vi "Network Settings Viewer_.vi"() -> ()   [LabVIEW 2015]
doc: "Displays network settings for network adapters on specified target. Target must have \"NI System Configuration Remote Support\" installed to correctly obtain all settings."
uses:
  <vilib>/nisyscfg/Access Point.ctl
  <vilib>/nisyscfg/Wireless Network.ctl
  <vilib>/Utility/error.llb/DialogType.ctl
  <vilib>/nisyscfg/Close (Hardware).vi
  <vilib>/nisyscfg/Close (Filter).vi
  <vilib>/nisyscfg/Close (System).vi
  <vilib>/nisyscfg/nisyscfg.lvlib
  <resource>/objmgr/nisysapi.rc
panel:
  in  "Timeout (milliseconds)":u32=5000
  in  "User Name":string
  in  "Password":string
  in  "Target":refnum<k21>="localhost"
  in  "Network Settings":enum32{"Ethernet", "WLAN", "WLAN Access Points"}(tab)
  out "Ethernet":string[][](table)
  out "WLAN":string[][](table) caption="Ethernet"
  out "Access Points":T1[](array[typedef]) {"wireless network"."security type" items=["none"=0, "open"=2, "WEP"=4, "WPA Personal"=8, "WPA Enterprise"=16, "WPA2 Personal"=32, "WPA2 Enterprise"=64]; "wireless network"."connection type" items=["none", "infrastructure", "ad hoc"]; "link speed" items=["none"=0, "autonegotiate"=1, "10mbps/Half Duplex"=2, "10mbps/Full Duplex"=4, "100mbps/Half Duplex"=8, "100mbps/Full Duplex"=16, "Gigabit/Half Duplex"=32, "Gigabit/Full Duplex"=64, "WLAN 802.11a"=131072, "WLAN 802.11b"=262144, "WLAN 802.11g"=524288, "WLAN 802.11n"=1048576, "WLAN 802.11n (5GHz)"=2097152]}
  # "Overview: Displays network settings for network adapters on specified target.\nRequirements: NI System Configuration\nInstructions:\n1. Select Target. Enter User Name and Password if necessary.\n2. Run the VI."
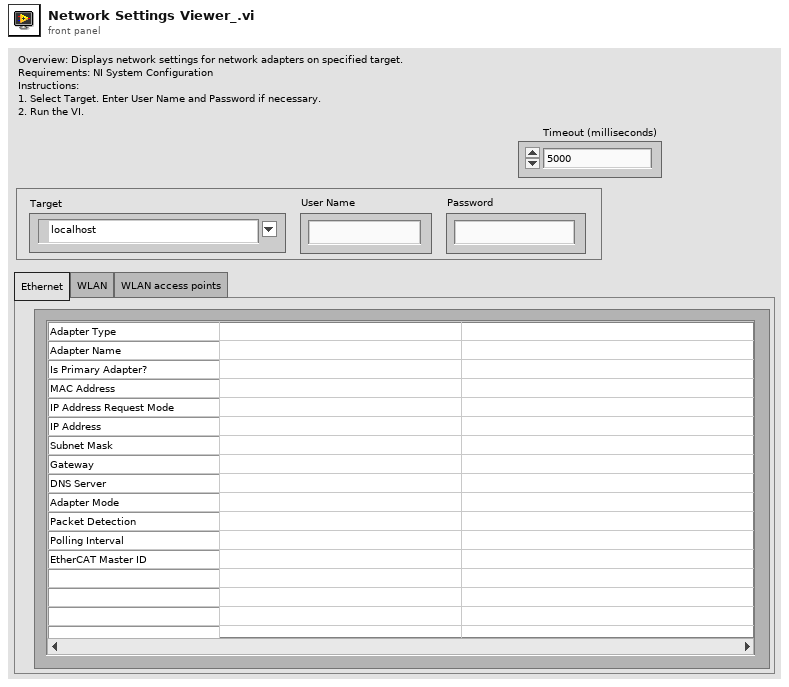
[diagram p1: front panel]
types:
  T1 = typedef "nisyscfg.lvlib/Access Point.ctl" = cluster{"wireless network":T2, "BSSID":string, "link quality":u32, "channel number":u32, "link speed":u32}
  T2 = typedef "nisyscfg.lvlib/Wireless Network.ctl" = cluster{"SSID":string, "connection type":u32, "security type":u32}
  T3 = typedef "DialogType.ctl" = u16
  T4 = typedef "Access Point.ctl" = cluster{"wireless network":T2, "BSSID":string, "link quality":u32, "channel number":u32, "link speed":u32}
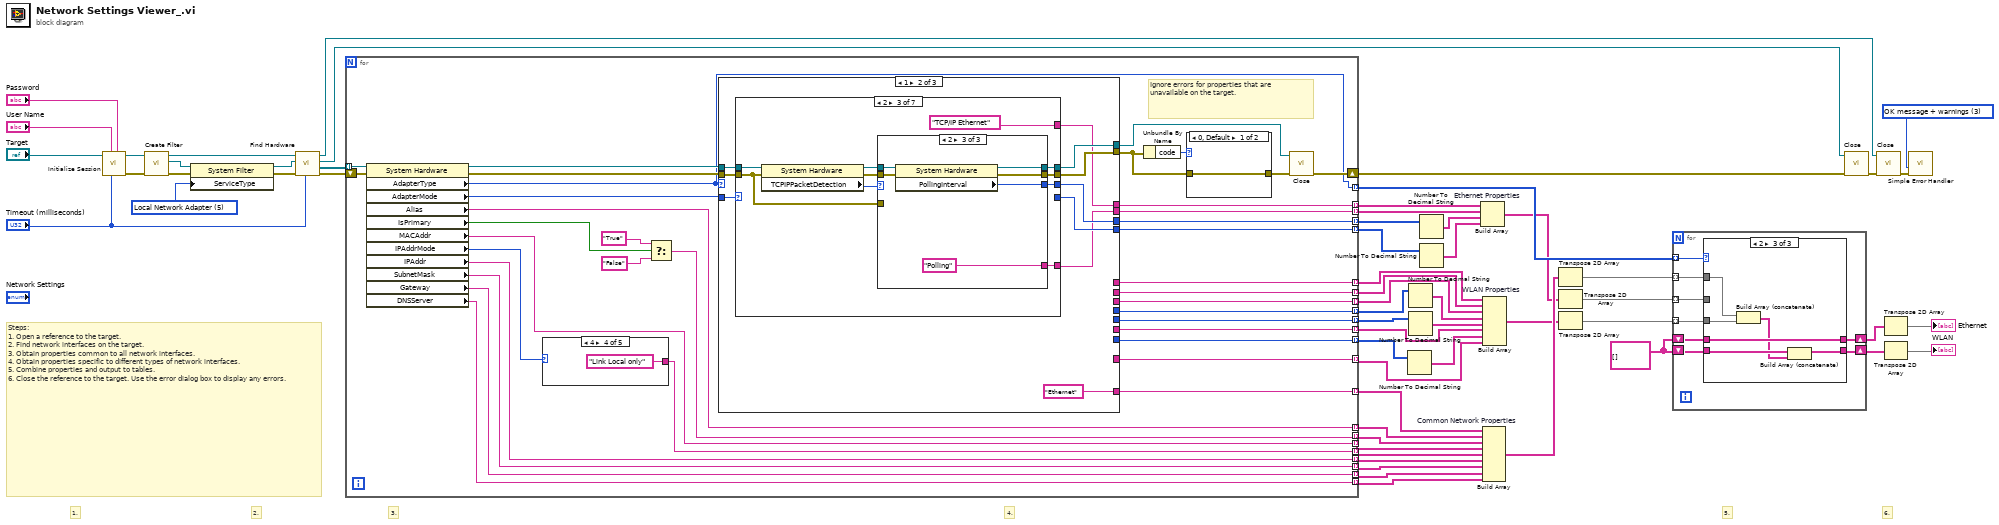
[diagram p0: block diagram]
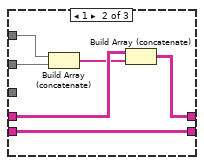
[diagram p3: hidden frame]
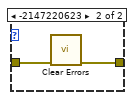
[diagram p4: hidden frame]
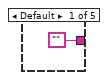
[diagram p5: hidden frame]
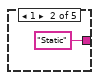
[diagram p6: hidden frame]
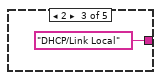
[diagram p7: hidden frame]
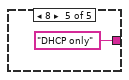
[diagram p8: hidden frame]
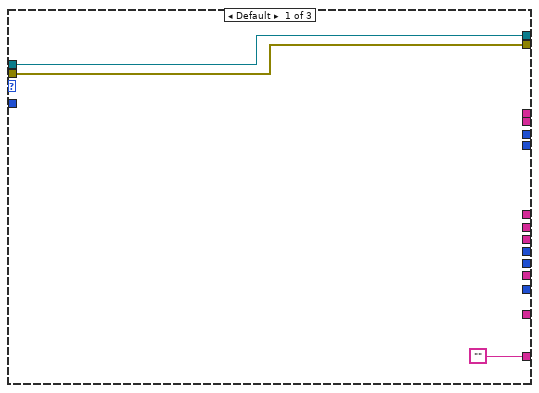
[diagram p9: hidden frame]
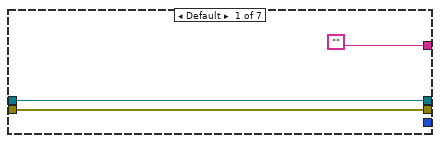
[diagram p10: hidden frame]
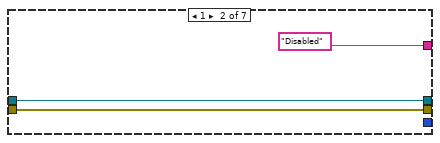
[diagram p11: hidden frame]
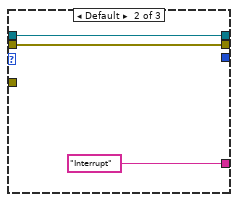
[diagram p13: hidden frame]
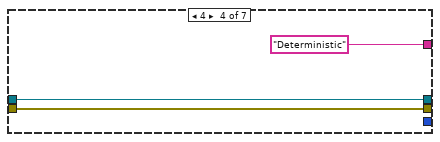
[diagram p14: hidden frame]
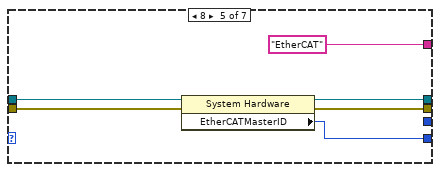
[diagram p15: hidden frame]
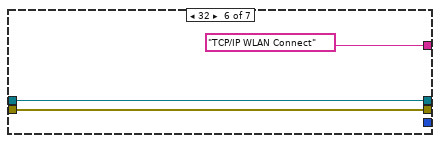
[diagram p16: hidden frame]
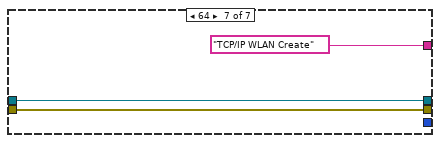
[diagram p17: hidden frame]
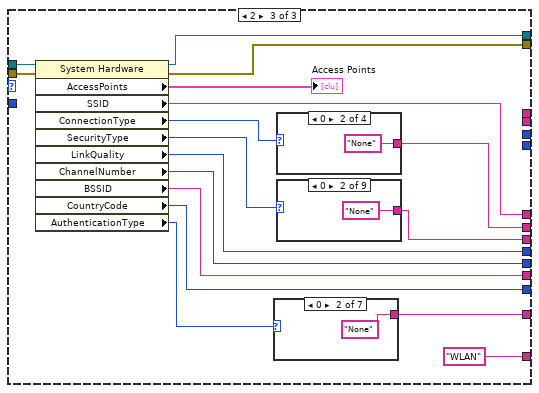
[diagram p18: hidden frame]
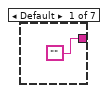
[diagram p19: hidden frame]
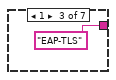
[diagram p20: hidden frame]
diagram:
  w3 = u32 5 items=["NI Network Resource", "NI Real-Time", "NI System Configuration", "NI Web Interface", "Local System", "Local Network Adapter", "Local Time Keeper", "Local Time Reference", "LXI Instrument"] ("Service Type")
  w4 = string[][] []
  w11 = T3 3 items=["no dialog", "OK message", "continue or stop message", "OK message + warnings", "continue/stop + warnings"] ("type of dialog (OK msg:1)")
  # "3."
  # "Steps:\n1. Open a reference to the target.\n2. Find network interfaces on the target.\n3. Obtain properties common to all network interfaces.\n4. Obtain properties specific to different types of network interfaces.\n5. Combine properties and output to tables.\n6. Close the reference to the target. Use the error dialog box to display any errors."
  # "6."
  # "5."
  # "4."
  # "2."
  # "1."
  n1 = call <vilib>:"Initialize Session.vi"("Password"="Password", "Connect Timeout (4000 ms)"="Timeout (milliseconds)", "User Name"="User Name", "Target (localhost)"="Target") -> ("error out"=w57:errorcluster, "Session out"=w58:refnum<k21>)  [unwired: 6 in]
  n2 = call <vilib>:"Create Filter.vi"("error in (no error)"=w57, "Session in"=w58) -> ("error out"=w55:errorcluster, "Filter out"=w56:refnum<k20>, "Session out"=w53:refnum<k21>)  [unwired: 7 in]
  n3 = property class="System Filter"(reference=w56, error in=w55, "ServiceType"=w3) -> (reference out=w52:refnum<k20>, error out=w54:errorcluster)
  n4 = call <vilib>:"Find Hardware.vi"("Remote Timeout (300,000 ms)"="Timeout (milliseconds)", "error in (no error)"=w54, "Filter in"=w52, "Session in"=w53) -> ("error out"=w51:errorcluster, "Resources out"=w10:refnum<k20>[], "Filter out"=w47:refnum<k20>, "Session out"=w48:refnum<k21>)  [unwired: 4 in]
  n5 = for {
    tunnel: w10 -> [w93] mode=indexing
    shift-right: [w92] -> w50
    shift-left: w51 -> [w94]
    tunnel: [w84] -> w45 mode=indexing
    tunnel: [w83] -> w44 mode=indexing
    tunnel: [w82] -> w43 mode=indexing
    tunnel: [w61] -> w42 mode=indexing
    tunnel: [w81] -> w41 mode=indexing
    tunnel: [w80] -> w40 mode=indexing
    tunnel: [w79] -> w39 mode=indexing
    tunnel: [w78] -> w22 mode=indexing
    tunnel: [w77] -> w24 mode=indexing
    tunnel: [w76] -> w25 mode=indexing
    tunnel: [w75] -> w31 mode=indexing
    tunnel: [w74] -> w32 mode=indexing
    tunnel: [w73] -> w28 mode=indexing
    tunnel: [w72] -> w29 mode=indexing
    tunnel: [w71] -> w30 mode=indexing
    tunnel: [w70] -> w2 mode=indexing
    tunnel: [w69] -> w38 mode=indexing
    tunnel: [w68] -> w37 mode=indexing
    tunnel: [w67] -> w35 mode=indexing
    tunnel: [w66] -> w34 mode=indexing
    tunnel: [w65] -> w21 mode=indexing
    tunnel: [w59] -> w1 mode=indexing
    # "Ignore errors for properties that are unavailable on the target."
    n6 = property class="System Hardware"(reference=w93, error in=w94) -> (reference out=w91:refnum<k20>, error out=w90:errorcluster, "AdapterType"=w65:u32, "AdapterMode"=w85:u32, "Alias"=w59:string, "IsPrimary"=w60:bool, "MACAddr"=w83:string, "IPAddrMode"=w86:u32, "IPAddr"=w61:string, "SubnetMask"=w81:string, "Gateway"=w80:string, "DNSServer"=w79:string)
    n7 = case "L10n_DhcpLinkLocal" shown="4" w86 {
      tunnel: ["" "Static" ("L10n_Static") "DHCP/Link Local" "Link Local only" ("L10n_LinkLocalOnly") "DHCP only" ("L10n_DhcpOnly")] -> w82
      frame Default {
      }
      frame 1 {
      }
      frame 2 {
      }
      frame 4 {
      }
      frame 8 {
      }
    }
    n8 = Select(t="True", s=w60, f="False") -> (s? t:f=w84:string)
    n9 = case shown="1" w65 {
      tunnel: w91 -> [w104 w115 w174]
      tunnel: w90 -> [w105 w114 w173]
      tunnel: [w105 w113 w167] -> w63
      tunnel: [w104 w112 w172] -> w89
      tunnel: w85 -> [_ w111 _]
      tunnel: ["" "Ethernet" ("L10n_TypeEthernet") "WLAN" ("L10n_TypeWlan")] -> w70
      tunnel: [_ w109 _] -> w67
      tunnel: [_ w108 _] -> w66
      tunnel: [_ w107 _] -> w69
      tunnel: [_ w106 _] -> w68
      tunnel: [_ _ w166] -> w71
      tunnel: [_ _ w165] -> w72
      tunnel: [_ _ w164] -> w73
      tunnel: [_ _ w163] -> w74
      tunnel: [_ _ w162] -> w75
      tunnel: [_ _ w161] -> w76
      tunnel: [_ _ w160] -> w77
      tunnel: [_ _ w159] -> w78
      frame Default {
      }
      frame 1 {
        n10 = case "L10n_ModeTcpipWlanConnect" shown="2" w111 {
          tunnel: w115 -> [w118 w120 w131 w143 w150 w152 w156]
          tunnel: w114 -> [w117 w119 w122 w144 w151 w153 w155]
          tunnel: [w117 w119 w127 w144 w149 w153 w155] -> w113
          tunnel: [w118 w120 w128 w143 w148 w152 w156] -> w112
          tunnel: ["" "Disabled" ("L10n_ModeDisabled") "TCP/IP Ethernet" ("L10n_ModeTcpipEthernet") "Deterministic" ("L10n_ModeDeterministic") "EtherCAT" ("L10n_ModeEtherCat") "TCP/IP WLAN Connect" "TCP/IP WLAN Create" ("L10n_ModeTcpipWlanCreate")] -> w107
          tunnel: [_ _ w124 _ _ _ _] -> w109
          tunnel: [_ _ _ _ w146 _ _] -> w108
          tunnel: [_ _ w123 _ _ _ _] -> w106
          frame Default {
          }
          frame 1 {
          }
          frame 2 {
            n11 = property class="System Hardware"(reference=w131, error in=w122) -> (reference out=w129:refnum<k20>, error out=w130:errorcluster, "TCPIPPacketDetection"=w126:u32)
            n12 = case shown="2" w126 {
              tunnel: w130 -> [_ w135 w141]
              tunnel: w129 -> [w132 w136 w142]
              tunnel: [w132 w136 w140] -> w128
              tunnel: [w133 w135 w139] -> w127
              tunnel: [_ "Interrupt" ("L10n_PacketInterrupt") "Polling" ("L10n_PacketPolling")] -> w123
              tunnel: [_ _ w137] -> w124
              tunnel: w122 -> [w133 _ _]
              frame 0 {
                # "Ignore errors here. May not support packet detection."
              }
              frame Default {
              }
              frame 2 {
                n13 = property class="System Hardware"(reference=w142, error in=w141) -> (reference out=w140:refnum<k20>, error out=w139:errorcluster, "PollingInterval"=w137:u32)
              }
            }
          }
          frame 4 {
          }
          frame 8 {
            n14 = property class="System Hardware"(reference=w150, error in=w151) -> (reference out=w148:refnum<k20>, error out=w149:errorcluster, "EtherCATMasterID"=w146:u32)
          }
          frame 32 {
          }
          frame 64 {
          }
        }
      }
      frame 2 {
        n15 = property class="System Hardware"(reference=w174, error in=w173) -> (reference out=w172:refnum<k20>, error out=w167:errorcluster, "AccessPoints"=→"Access Points":T4[], "SSID"=w166:string, "ConnectionType"=w170:u32, "SecurityType"=w169:u32, "LinkQuality"=w163:u32, "ChannelNumber"=w162:u32, "BSSID"=w161:string, "CountryCode"=w160:i32, "AuthenticationType"=w168:u32)
        n16 = case shown="0" w168 {
          tunnel: ["" "None" ("L10n_AuthNone") "EAP-TLS" "EAP-TTLS" "EAP-FAST" "LEAP" "PEAP"] -> w159
          frame Default {
          }
          frame 0 {
          }
          frame 1 {
          }
          frame 2 {
          }
          frame 4 {
          }
          frame 8 {
          }
          frame 16 {
          }
        }
        n17 = case shown="0" w170 {
          tunnel: ["" "None" ("L10n_ConnNone") "Infrastructure" ("L10n_ConnInfrastructure") "Ad Hoc" ("L10n_ConnAdHoc")] -> w165
          frame Default {
          }
          frame 0 {
          }
          frame 1 {
          }
          frame 2 {
          }
        }
        n18 = case shown="0" w169 {
          tunnel: ["" "None" ("L10n_SecurityNone") "Not Supported" ("L10n_SecurityNotSupported") "Open" ("L10n_SecurityOpen") "WEP" "WPA-PSK" "WPA-EAP" "WPA2-PSK" "WPA2-EAP"] -> w164
          frame Default {
          }
          frame 0 {
          }
          frame 1 {
          }
          frame 2 {
          }
          frame 4 {
          }
          frame 8 {
          }
          frame 16 {
          }
          frame 32 {
          }
          frame 64 {
          }
        }
      }
    }
    n19 = Unbundle By Name(w63) -> ("code"=w64:i32)
    n20 = case shown="0, Default" w64 {
      tunnel: [w95 w97] -> w62
      tunnel: w63 -> [w95 w96]
      frame 0, Default {
      }
      frame -2147220623 {
        n21 = call <vilib>:"Clear Errors.vi"("error in (no error)"=w96) -> ("error out"=w97:errorcluster)  [unwired: 5 in, 1 out]
      }
    }
    n22 = call-poly <vilib>:"Close.vi"("error in (no error)"=w62, "Resource in"=w89) -> ("error out"=w92:errorcluster)  [unwired: 9 in]
  }
  n23 = Number To Decimal String(number=w24) -> (decimal integer string=w23:string[])  [unwired: 1 in]
  n24 = Number To Decimal String(number=w32) -> (decimal integer string=w27:string[])  [unwired: 1 in]
  n25 = Number To Decimal String(number=w31) -> (decimal integer string=w26:string[])  [unwired: 1 in]
  n26 = Number To Decimal String(number=w35) -> (decimal integer string=w33:string[])  [unwired: 1 in]
  n27 = Number To Decimal String(number=w34) -> (decimal integer string=w36:string[])  [unwired: 1 in]
  n28 = Build Array "Ethernet Properties"(w38, w37, w33, w36) -> (w18:string[][])
  n29 = Build Array "Common Network Properties"(w2, w1, w45, w44, w43, w42, w41, w40, w39) -> (w20:string[][])
  n30 = Build Array "WLAN Properties"(w30, w29, w28, w27, w26, w25, w23, w22) -> (w14:string[][])
  n31 = Transpose 2D Array(2D array=w20) -> (transposed array=w19:string[][])
  n32 = Transpose 2D Array(2D array=w18) -> (transposed array=w17:string[][])
  n33 = Transpose 2D Array(2D array=w14) -> (transposed array=w13:string[][])
  n34 = for {
    tunnel: w21 -> [w199] mode=indexing
    tunnel: w19 -> [w201] mode=indexing
    tunnel: w17 -> [w202] mode=indexing
    tunnel: w13 -> [w198] mode=indexing
    shift-right: [w197] -> w15
    shift-left: w4 -> [w196]
    shift-right: [w200] -> w16
    shift-left: w4 -> [w195]
    n35 = case shown="2" w199 {
      tunnel: w202 -> [_ w208 _]
      tunnel: w201 -> [_ w207 w214]
      tunnel: [_ w203 w210] -> w200
      tunnel: w198 -> [_ _ w213]
      tunnel: [_ w206 w212] -> w197
      tunnel: w196 -> [_ w206 w211]
      tunnel: w195 -> [_ w205 w210]
      frame Default {
      }
      frame 1 {
        n36 = Build Array (concatenate)(w207, w208) -> (w204:string[])
        n37 = Build Array (concatenate)(w205, w204) -> (w203:string[][])
      }
      frame 2 {
        n38 = Build Array (concatenate)(w214, w213) -> (w209:string[])
        n39 = Build Array (concatenate)(w211, w209) -> (w212:string[][])
      }
    }
  }
  n40 = call-poly <vilib>:"Close.vi"("error in (no error)"=w50, "Filter in"=w47) -> ("error out"=w49:errorcluster)  [unwired: 9 in]
  n41 = call-poly <vilib>:"Close.vi"("error in (no error)"=w49, "Session in"=w48) -> ("error out"=w46:errorcluster)  [unwired: 9 in]
  n42 = Transpose 2D Array(2D array=w16) -> (transposed array=→"Ethernet":string[][])
  n43 = Transpose 2D Array(2D array=w15) -> (transposed array=→"WLAN":string[][])
  n44 = call <vilib>:"Simple Error Handler.vi"("type of dialog (OK msg:1)"=w11, "error in (no error)"=w46) -> ()  [unwired: 3 in, 5 out]
